vi "ConvertStringTimeToSecond.vi"(8 "e-load 제어 딜레이 때문에 추가":bool, 11 "StringTime":string) -> (3 "Second":dbl)   [LabVIEW 2018, in "Library-DataConvert.lvlib"]
uses:
  Library-DataConvert.lvlib
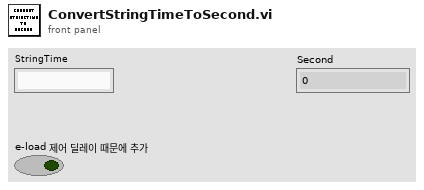
[diagram p1: front panel]
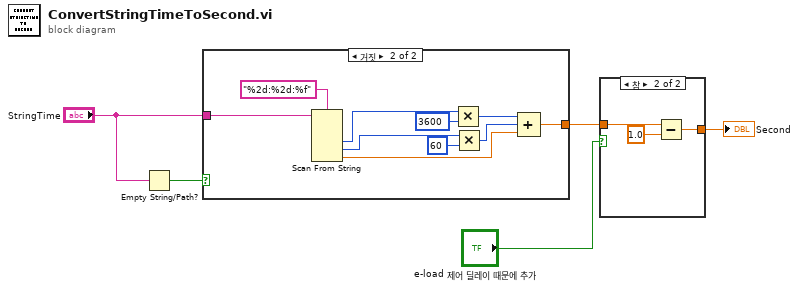
[diagram p0: block diagram]
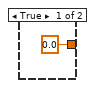
[diagram p3: hidden frame]
diagram:
  n1 = Empty String/Path?(string/path="StringTime") -> (empty?=w4:bool)
  n2 = case shown="거짓" w4 {
    tunnel: [0.0 w8] -> w5
    tunnel: "StringTime" -> [_ w7]
    frame True {
    }
    frame False {
      n3 = Scan From String(format string="%2d:%2d:%f" ("포맷 문자열"), input string=w7) -> (output 1=w15:i32, output 2=w13:i32, output 3=w9:dbl)  [unwired: 5 in, 3 out]
      n4 = Multiply(x=w15, y=3600) -> (x*y=w11:i32)
      n5 = Multiply(x=w13, y=60) -> (x*y=w10:i32)
      n6 = Compound Arithmetic op=ADD(w11, w10, w9) -> (w8:dbl)
    }
  }
  n7 = case shown="참" "e-load 제어 딜레이 때문에 추가" {
    tunnel: w5 -> [w17 w20]
    tunnel: [w17 w19] -> w2
    frame False {
    }
    frame True {
      n8 = Subtract(x=w20, y=1.0) -> (x-y=w19:dbl)
    }
  }
  "Second" <- w2
